vi "GetActualValues.vi"(7 "LabVIEW Web Service Request":refnum<class "Web Request.lvclass">) -> ()   [LabVIEW 2019]
uses:
  <vilib>/wsapi/Web Request.lvclass
  WebServiceData_class/WebServiceData.lvclass
panel:
  # "Use the Web Service Request input terminal to call the VIs on the Web Services palette. Do not remove it from the connector pane unless you don't need access to the palette."
  # "Each additional control wired to the connector pane will be available as an input in the URL. To include an indicator in terminal-mode output (the default setting), it must also be wired to the connector pane."
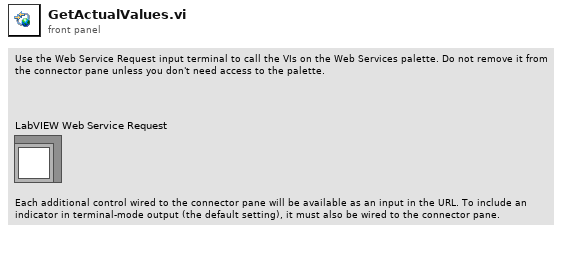
[diagram p1: front panel]
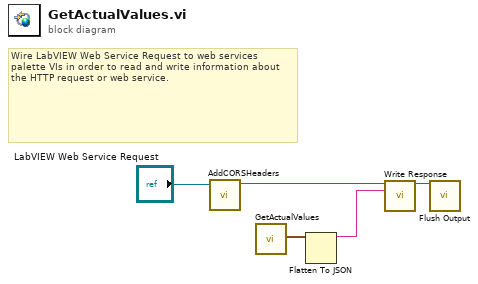
[diagram p0: block diagram]
diagram:
  # "Wire LabVIEW Web Service Request to web services palette VIs in order to read and write information about the HTTP request or web service."
  n1 = call "AddCORSHeaders.vi"("LabVIEW Web Service Request"="LabVIEW Web Service Request") -> ("LabVIEW Web Service Request out"=w2:refnum<class "Web Request.lvclass">)  [unwired: 9 in, 1 out]
  n2 = call "GetActualValues.vi"() -> ("ActualValues"=w4:cluster{"T":dbl, "RH":dbl})  [unwired: 18 in, 1 out]
  n3 = Flatten To JSON(anything=w4) -> (JSON string=w1:string)  [unwired: 2 in, 1 out]
  n4 = call <vilib>:"Write Response.vi"("LabVIEW Web Service Request"=w2, "response string"=w1) -> ("LabVIEW Web Service Request out"=w3:refnum<class "Web Request.lvclass">)  [unwired: 12 in, 1 out]
  n5 = call <vilib>:"Flush Output.vi"("LabVIEW Web Service Request"=w3) -> ()  [unwired: 13 in, 2 out]
